vi "MapCoordinates_SUBVI.vi"(11 "Mouse":T1) -> (3 "Pulse Width Array":u16[](array[numeric]))   [LabVIEW 2020]
uses:
  <vilib>/Utility/miscctls.llb/LVMouseTypeDef.ctl
  <vilib>/Analysis/NI_AALPro.lvlib
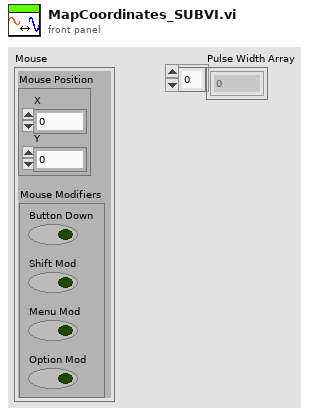
[diagram p1: front panel]
types:
  T1 = typedef "LVMouseTypeDef.ctl" = cluster{"Mouse Position":cluster{"X":i32, "Y":i32}, "Mouse Modifiers":cluster{"Button Down":bool, "Shift Mod":bool, "Menu Mod":bool, "Option Mod":bool}}
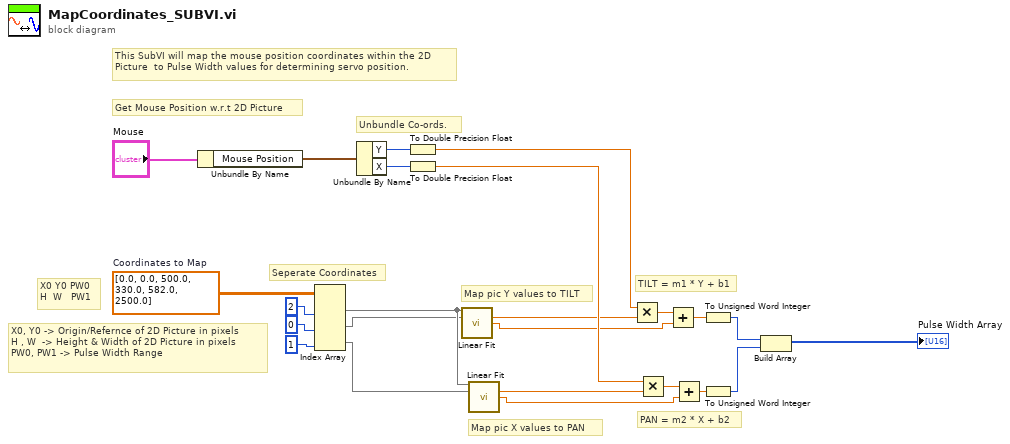
[diagram p0: block diagram]
diagram:
  w21 = dbl[][] [[0.0, 0.0, 500.0], [330.0, 582.0, 2500.0]]  # Coordinates to Map
  # "X0 Y0 PW0\nH  W   PW1"
  # "X0, Y0 -> Origin/Refernce of 2D Picture in pixels\nH , W  -> Height & Width of 2D Picture in pixels\nPW0, PW1 -> Pulse Width Range"
  # "PAN = m2 * X + b2"
  # "TILT = m1 * Y + b1"
  # "Map pic Y values to TILT"
  # "Map pic X values to PAN"
  # "This SubVI will map the mouse position coordinates within the 2D Picture  to Pulse Width values for determining servo position."
  # "Seperate Coordinates"
  # "Unbundle Co-ords."
  # "Get Mouse Position w.r.t 2D Picture"
  n1 = Unbundle By Name("Mouse") -> ("Mouse Position"=w7:cluster{"X":i32, "Y":i32})
  n2 = Index Array(array=w21, index (col) #1=2 ("index (row)"), index (col) #2=0 ("index (row)"), index (col) #3=1 ("index (col)")) -> (element #1=w22:dbl[], element #2=w2:dbl[], element #3=w6:dbl[])  [unwired: 3 in]
  n3 = Unbundle By Name(w7) -> ("Y"=w8:i32, "X"=w17:i32)
  n4 = To Double Precision Float(number=w8) -> (double precision float=w10:dbl)
  n5 = To Double Precision Float(number=w17) -> (double precision float=w18:dbl)
  n6 = call <vilib>:"Linear Fit.vi"("Y"=w22, "X"=w2) -> ("slope"=w9:dbl, "intercept"=w12:dbl)  [unwired: 9 in, 3 out]
  n7 = call <vilib>:"Linear Fit.vi"("Y"=w22, "X"=w6) -> ("slope"=w19:dbl, "intercept"=w16:dbl)  [unwired: 9 in, 3 out]
  n8 = Multiply(x=w10, y=w9) -> (x*y=w11:dbl)
  n9 = Multiply(x=w18, y=w19) -> (x*y=w15:dbl)
  n10 = Add(x=w11, y=w12) -> (x+y=w13:dbl)
  n11 = Add(x=w15, y=w16) -> (x+y=w14:dbl)
  n12 = To Unsigned Word Integer(number=w13) -> (unsigned 16bit integer=w23:u16)
  n13 = To Unsigned Word Integer(number=w14) -> (unsigned 16bit integer=w24:u16)
  n14 = Build Array(w23, w24) -> (→"Pulse Width Array":u16[])
